vi "LED_State.vi"(8 "error in (no error)":errorcluster) -> (0 "error out":errorcluster, 2 "Red LED State":bool, 3 "Green LED State":bool)   [LabVIEW 2014]
uses:
  <userlib>/UCSD Robotics Lab/Robotics-Cape/LV/libroboticscape.lvlib
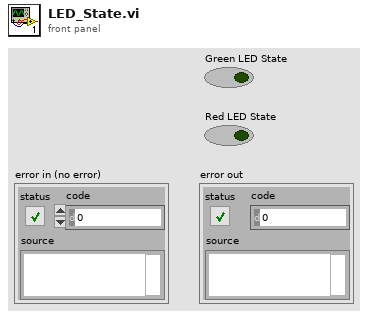
[diagram p1: front panel]
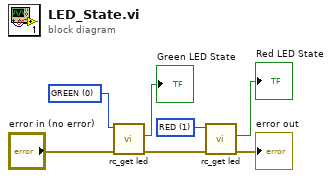
[diagram p0: block diagram]
diagram:
  w3 = u32 1 items=["GREEN", "RED"] ("led")
  w1 = u32 0 items=["GREEN", "RED"] ("led")
  n1 = call <userlib>:"rc_get led.vi"("error in (no error)"="error in (no error)", "led"=w1) -> ("error out"=w2:errorcluster, "LED On/Off"=→"Green LED State":bool)  [unwired: 7 in, 1 out]
  n2 = call <userlib>:"rc_get led.vi"("error in (no error)"=w2, "led"=w3) -> ("error out"=→"error out":errorcluster, "LED On/Off"=→"Red LED State":bool)  [unwired: 7 in, 1 out]
